vi "AutoHelper_Sequence.vi"(4 "Next Step":bool, 6 "Pass_Through_Time":dbl=-1.0 format="%33.4f", 7 "External Ready":bool=TRUE, 8 "Cancel Time Sec":dbl, 9 "Step Times Sec":dbl[](array[numeric]), 10 "Cancel":bool, 11 "Initiate":bool) -> (0 "Error":bool, 1 "Ready":bool, 2 "Seq  Active":bool, 3 "Step Number":T1=enum."Initialize", 5 "New Step":bool)   [LabVIEW 2019, in "Trajectory_Library.lvlib"]
doc: "Implements a simplified state machine similar to a mechanical / electrical drum sequencer. When the Drum Sequencer is \"Ready\" and the \"Initiate\" input becomes TRUE,, the drum sequences through its set of steps from 1 to N. After each Step is executed it is followed by a wait. During the wait the Step output indicates \"Do Nothing\". The number of Steps is determined by the number of elements in the \"Step Times\" input array. Once all the steps have been executed, the Drum Sequencer cycles bac to wait for another initiate. \n\nThere is a Cancel input that interrupts the sequence, executes the Cancel Step, performs the cancel wait, and then returns to wait for an Initiate action. \n\nIf any of the Step Times, or Cancel times are negative, or there more than 32 steps, or less than 1 step an error is signaled. The drum sequencer selects the error state and stays there.\n\nInputs:\n\nOutputs:"
uses:
  Trajectory_Library.lvlib
  Enum/DrumSequence_Step_Enum.ctl
  Enum/DrumSequence_State_Enum.ctl
  Util_GetTime_U32.vi
  Util_GetTime_U64.vi
  <vilib>/Utility/semaphor.llb/Obtain Semaphore Reference.vi
  Timer_Reset.vi
panel:
  # "Time to wait\nafter executing\nstep"
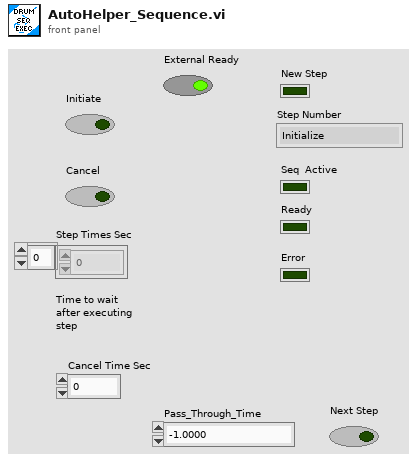
[diagram p1: front panel]
types:
  T1 = typedef "Trajectory_Library.lvlib/DrumSequence_Step_Enum.ctl" = enum16{"Do Nothing", "Step 1", "Step 2", "Step 3", "Step 4", "Step 5", "Step 6", "Step 7", "Step 8", "Step 9", "Step 10", "Step 11", "Step 12", "Step 13", "Step 14", "Step 15", "Step 16", "Step 17", "Step 18", "Step 19", "Step 20", "Step 21", "Step 22", "Step 23", "Step 24", "Step 25", "Step 26", "Step 27", "Step 28", "Step 29", "Step 30", "Step 31", "Step 32", "Cancel", "Initialize", "Error"}
  T2 = typedef "Trajectory_Library.lvlib/DrumSequence_State_Enum.ctl" = enum16{"Initialize", "Ready", "First Step", "Step Wait", "Next State", "Cancel", "Cancel Wait", "Error", "Error Loop"}
  T3 = typedef "Trajectory_Library.lvlib/TIMER.ctl" = cluster{"StartTime":dbl, "Accumulated TIme":dbl, "Running":bool, "semaphore":T4}
  T4 = typedef "Semaphore RefNum" = refnum<k1>
  T5 = typedef "DrumSequence_State_Enum.ctl" = enum16{"Initialize", "Ready", "First Step", "Step Wait", "Next State", "Cancel", "Cancel Wait", "Error", "Error Loop"}
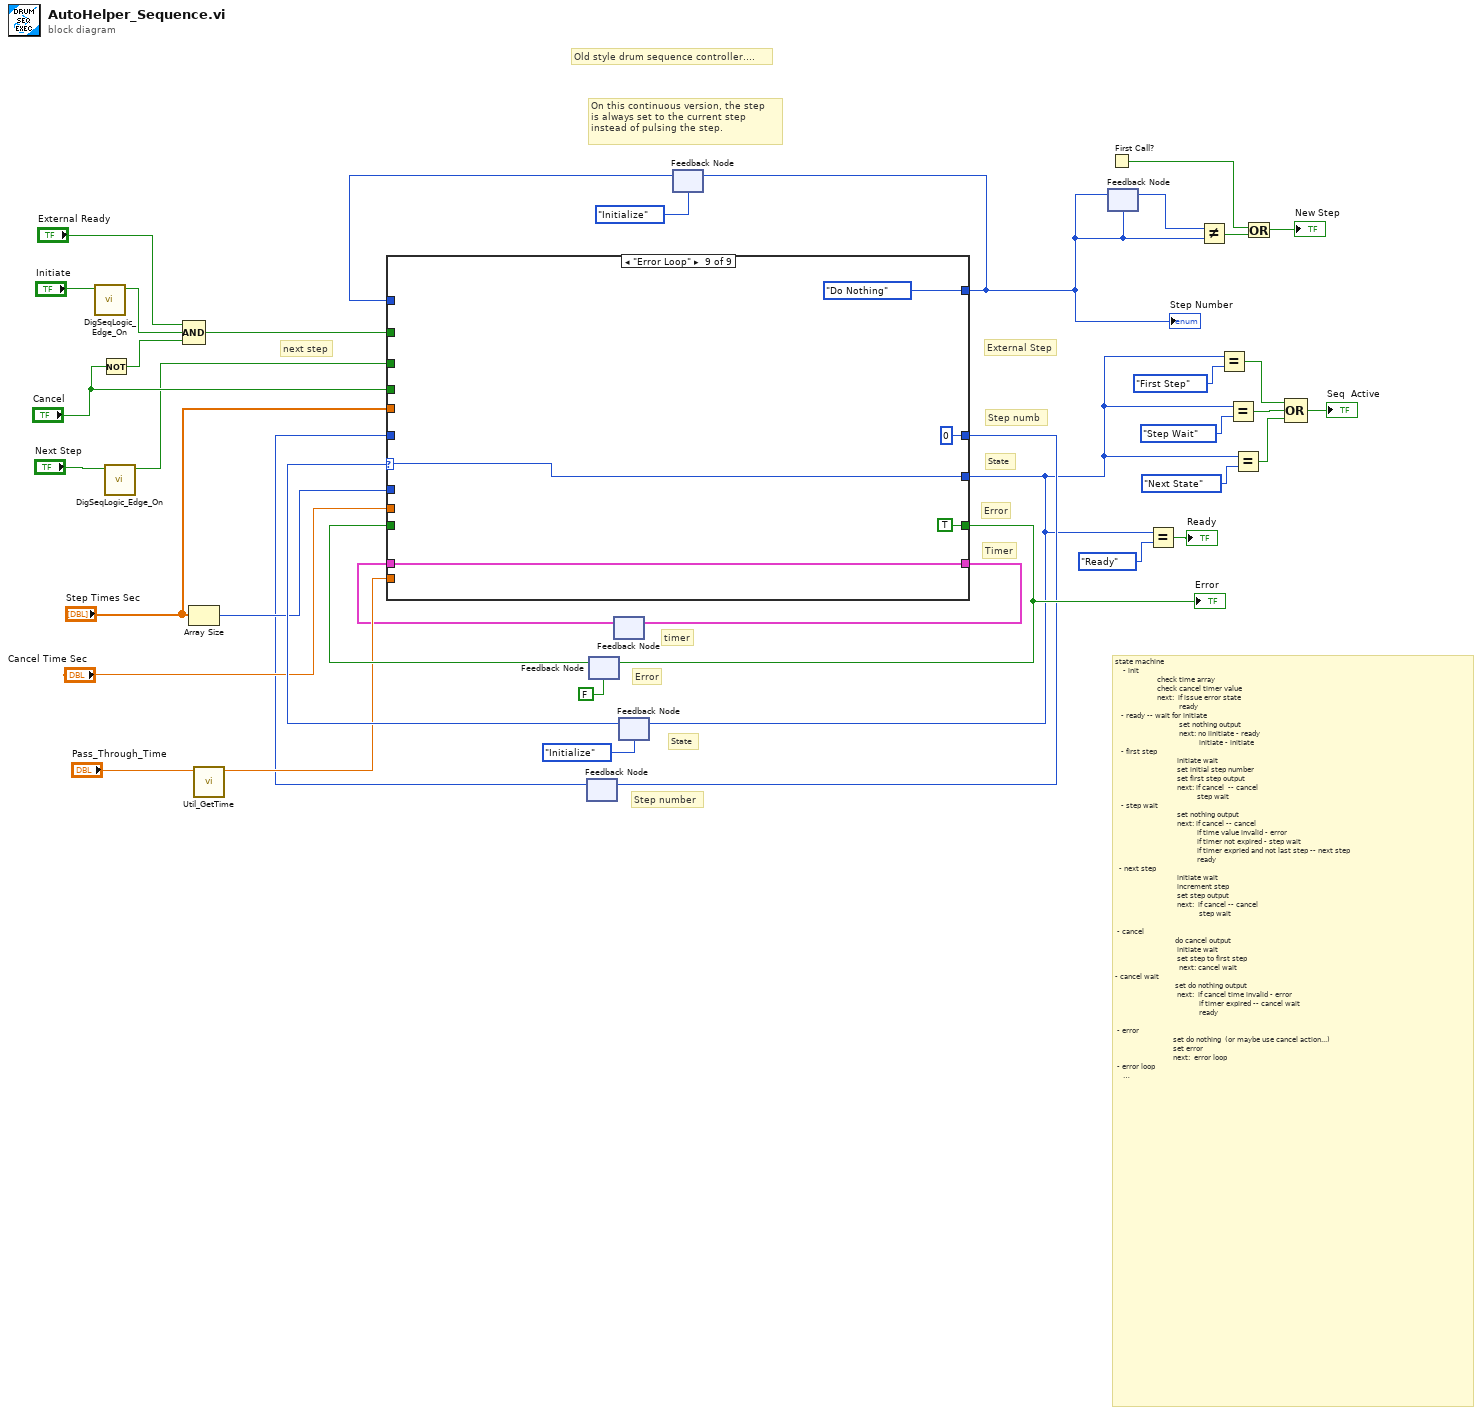
[diagram p0: block diagram]
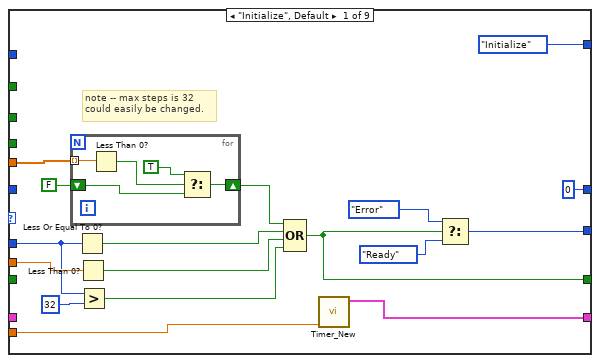
[diagram p2: hidden frame]
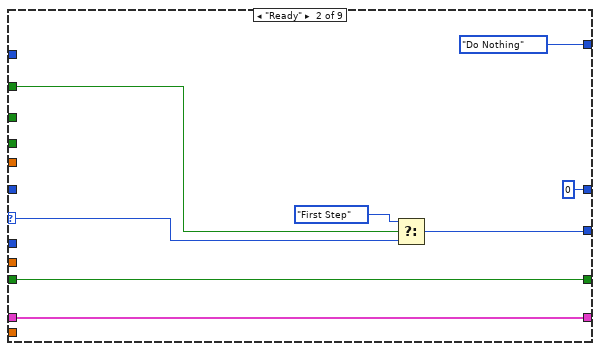
[diagram p3: hidden frame]
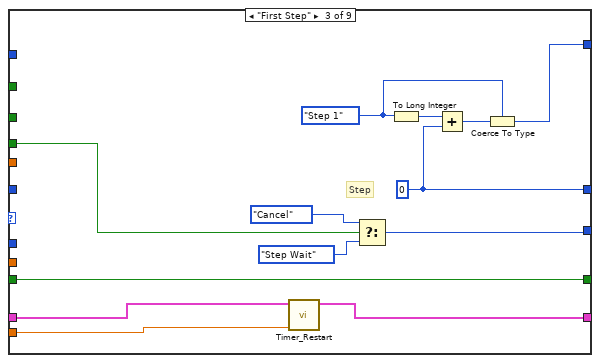
[diagram p4: hidden frame]
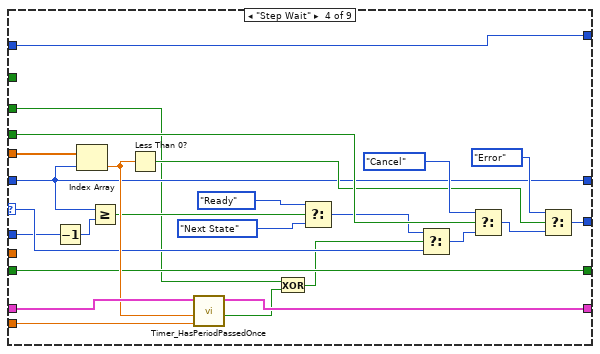
[diagram p5: hidden frame]
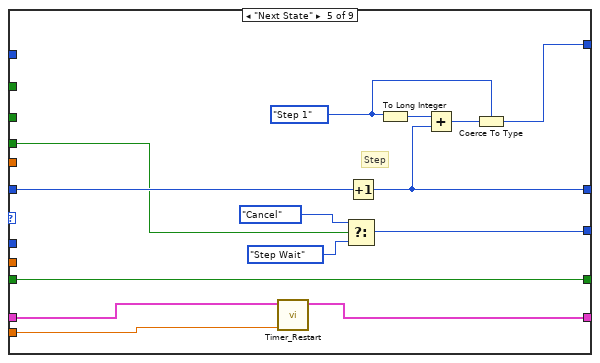
[diagram p6: hidden frame]
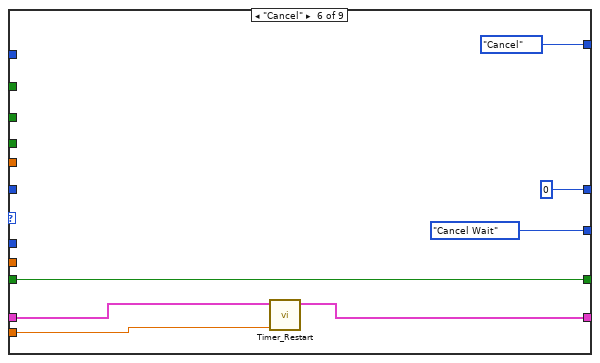
[diagram p7: hidden frame]
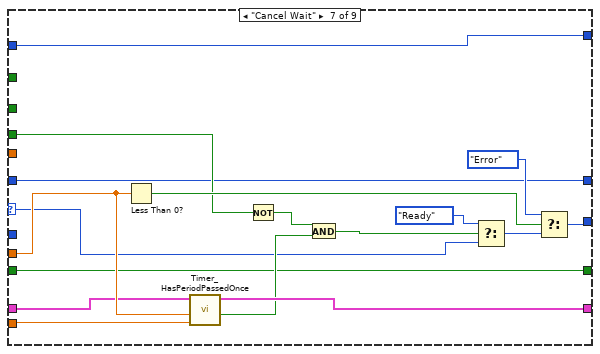
[diagram p8: hidden frame]
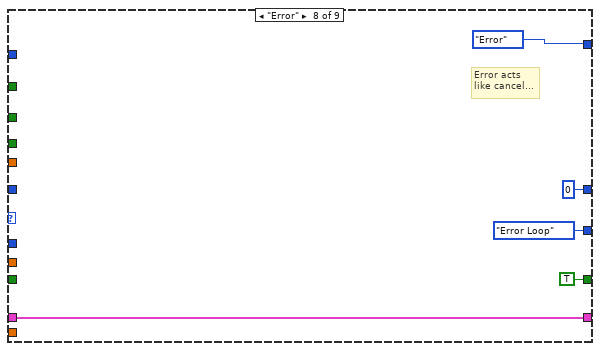
[diagram p9: hidden frame]
diagram:
  # "On this continuous version, the step\nis always set to the current step\ninstead of pulsing the step."
  # "next step"
  # "Old style drum sequence controller...."
  # "Step number"
  # "State"
  # "Step numb"
  # "timer"
  # "Timer"
  # "Error"
  # "State"
  # "External Step"
  # "Error"
  # "state machine\n    - init\n                     check time array\n                     check cancel timer value\n                     next:  if issue error state\n                                ready\n   - ready -- wait for initiate\n                                set nothing output\n                                next: no iinitiate - ready\n                                          initiate - initiate\n   - first step \n                               initiate wait\n                               set initial step number\n                               set first step output\n                               next: if cancel  -- cancel\n                                         step wait\n   - step wait \n                               set nothing output\n                               next: if cancel -- cancel\n                                         if time value invalid - error\n                                         if timer not expired - step wait\n                                         if timer expried and not last step -- next step\n                                         ready\n  - next step\n                               initiate wait\n                               increment step\n                               set step output\n                               next:  if cancel -- cancel\n                                          step wait\n\n - cancel\n                              do cancel output\n                               initiate wait\n                               set step to first step\n                                next: cancel wait\n- cancel wait\n                              set do nothing output\n                               next:  if cancel time invalid - error\n                                          if timer expired -- cancel wait\n                                          ready\n\n - error\n                             set do nothing  (or maybe use cancel action...)\n                             set error\n                             next:  error loop\n - error loop\n                             set do nothing\n                             set error\n                             next: error loop"
  n1 = call "DigSeqLogic_Edge_On.vi"("Input"="Initiate") -> ("On Edge"=w37:bool)  [unwired: 10 in]
  n2 = Not(x="Cancel") -> (.not. x?=w39:bool)
  n3 = call "DigSeqLogic_Edge_On.vi"("Input"="Next Step") -> ("On Edge"=w8:bool)  [unwired: 10 in]
  n4 = Compound Arithmetic op=AND("External Ready", w37, w39) -> (w26:bool)
  n5 = Array Size(array="Step Times Sec") -> (size(s)=w34:i32)
  n6 = call "Util_GetTime.vi"("Pass_Through_Time"="Pass_Through_Time") -> ("FPGA_Time_Seconds"=w27:dbl)  [unwired: 8 in, 2 out]
  n7 = feedback #1() -> (w20:i32)  [unwired: 1 in]
  n8 = feedback #2(FALSE) -> (w29:bool)
  n9 = feedback #3() -> (w19:T3)  [unwired: 1 in]
  n10 = feedback #4(DrumSequence_State_Enum."Initialize") -> (w35:T5)
  n11 = feedback #5(DrumSequence_Step_Enum."Initialize" ("Step Number")) -> (w1:T1)
  n12 = case shown="\"Error Loop\"" w35 {
    selector: w35 -> [_ w66 _ w90 _ _ w130 _ w154]
    tunnel: w34 -> [w44 _ _ w88 _ _ _ _ _]
    tunnel: "Step Times Sec" -> [w55 _ _ w98 _ _ _ _ _]
    tunnel: "Cancel Time Sec" -> [w54 _ _ _ _ _ w142 _ _]
    tunnel: [w50 w65 w71 w91 w112 w124 w131 TRUE TRUE] -> w30
    tunnel: w29 -> [_ w65 w71 w91 w112 w124 w131 _ _]
    tunnel: [w47 w67 w72 w95 w114 DrumSequence_State_Enum."Cancel Wait" w135 DrumSequence_State_Enum."Error Loop" w154] -> w11
    tunnel: [w46 w64 w76 w105 w109 w125 w139 w148 w152] -> w23
    tunnel: w27 -> [w45 _ w78 w106 w111 w126 w140 _ _]
    tunnel: [DrumSequence_Step_Enum."Initialize" ("Step Number") DrumSequence_Step_Enum."Do Nothing" ("Step Number") w80 w83 w115 DrumSequence_Step_Enum."Cancel" ("Step Number") w129 DrumSequence_Step_Enum."Error" ("Step Number") DrumSequence_Step_Enum."Do Nothing" ("Step Number")] -> w3
    tunnel: w26 -> [_ w69 _ _ _ _ _ _ _]
    tunnel: [0 0 w79 w92 w116 0 w133 0 0] -> w21
    tunnel: "Cancel" -> [_ _ w75 w102 w113 _ w136 _ _]
    tunnel: w20 -> [_ _ _ w92 w117 _ w133 _ _]
    tunnel: w19 -> [_ w64 w77 w107 w110 w127 w141 w148 w152]
    tunnel: w8 -> [_ _ _ w84 _ _ _ _ _]
    tunnel: w1 -> [_ _ _ w83 _ _ w129 _ _]
    frame "Initialize", Default {
      # "note -- max steps is 32\ncould easily be changed."
      n13 = for {
        shift-right: [w60] -> w53
        shift-left: FALSE -> [w59]
        tunnel: w55 -> [w61] mode=indexing
        n14 = Less Than 0?(x=w61) -> (x < 0?=w57:bool)
        n15 = Select(t=TRUE, s=w57, f=w59) -> (s? t:f=w60:bool)
      }
      n16 = Less Or Equal To 0?(x=w44) -> (x <= 0?=w52:bool)
      n17 = Less Than 0?(x=w54) -> (x < 0?=w51:bool)
      n18 = Greater?(x=w44, y=32) -> (0:w42:bool)
      n19 = Compound Arithmetic op=OR(w53, w52, w51, w42) -> (w50:bool)
      n20 = call "Timer_New.vi"("Pass_Through_Time"=w45) -> ("TIMER"=w46:T3)  [unwired: 10 in]
      n21 = Select(t=DrumSequence_State_Enum."Error", s=w50, f=DrumSequence_State_Enum."Ready") -> (s? t:f=w47:T2)
    }
    frame "Ready" {
      n22 = Select(t=DrumSequence_State_Enum."First Step", s=w69, f=w66) -> (s? t:f=w67:T5)
    }
    frame "First Step" {
      w70 = DrumSequence_Step_Enum."Step 1" ("Step Number")
      w79 = 0
      # "Step"
      n23 = call "Timer_Restart.vi"("Pass_Through_Time"=w78, "in Timer"=w77) -> ("out Timer"=w76:T3)  [unwired: 9 in]
      n24 = Select(t=DrumSequence_State_Enum."Cancel", s=w75, f=DrumSequence_State_Enum."Step Wait") -> (s? t:f=w72:T2)
      n25 = To Long Integer(number=w70) -> (32bit integer=w82:i32)
      n26 = Add(x=w82, y=w79) -> (x+y=w81:i32)
      n27 = Coerce To Type(0:w81, 1:w70) -> (2:w80:T1)
    }
    frame "Step Wait" {
      n28 = Decrement(x=w88) -> (x-1=w89:i32)
      n29 = Index Array(array=w98, index=w92) -> (element=w97:dbl)
      n30 = Greater Or Equal?(x=w92, y=w89) -> (x >= y?=w87:bool)
      n31 = Less Than 0?(x=w97) -> (x < 0?=w93:bool)
      n32 = call "Timer_HasPeriodPassedOnce.vi"("Pass_Through_Time"=w106, "Period"=w97, "in Timer"=w107) -> ("Expired"=w86:bool, "out Timer"=w105:T3)  [unwired: 6 in, 1 out]
      n33 = Exclusive Or(1:w86, 2:w84) -> (0:w85:bool)
      n34 = Select(t=DrumSequence_State_Enum."Ready", s=w87, f=DrumSequence_State_Enum."Next State") -> (s? t:f=w99:T2)
      n35 = Select(t=w99, s=w85, f=w90) -> (s? t:f=w103:T5)
      n36 = Select(t=DrumSequence_State_Enum."Cancel", s=w102, f=w103) -> (s? t:f=w94:T5)
      n37 = Select(t=DrumSequence_State_Enum."Error", s=w93, f=w94) -> (s? t:f=w95:T5)
    }
    frame "Next State" {
      w108 = DrumSequence_Step_Enum."Step 1" ("Step Number")
      # "Step"
      n38 = call "Timer_Restart.vi"("Pass_Through_Time"=w111, "in Timer"=w110) -> ("out Timer"=w109:T3)  [unwired: 9 in]
      n39 = Select(t=DrumSequence_State_Enum."Cancel", s=w113, f=DrumSequence_State_Enum."Step Wait") -> (s? t:f=w114:T2)
      n40 = Increment(x=w117) -> (x+1=w116:i32)
      n41 = To Long Integer(number=w108) -> (32bit integer=w121:i32)
      n42 = Add(x=w121, y=w116) -> (x+y=w120:i32)
      n43 = Coerce To Type(0:w120, 1:w108) -> (2:w115:T1)
    }
    frame "Cancel" {
      n44 = call "Timer_Restart.vi"("Pass_Through_Time"=w126, "in Timer"=w127) -> ("out Timer"=w125:T3)  [unwired: 9 in]
    }
    frame "Cancel Wait" {
      n45 = Less Than 0?(x=w142) -> (x < 0?=w143:bool)
      n46 = call "Timer_HasPeriodPassedOnce.vi"("Pass_Through_Time"=w140, "Period"=w142, "in Timer"=w141) -> ("Expired"=w138:bool, "out Timer"=w139:T3)  [unwired: 6 in, 1 out]
      n47 = Not(x=w136) -> (.not. x?=w137:bool)
      n48 = And(x=w137, y=w138) -> (x .and. y?=w132:bool)
      n49 = Select(t=DrumSequence_State_Enum."Ready", s=w132, f=w130) -> (s? t:f=w144:T5)
      n50 = Select(t=DrumSequence_State_Enum."Error", s=w143, f=w144) -> (s? t:f=w135:T5)
    }
    frame "Error" {
      # "Error acts\nlike cancel..."
    }
    frame "Error Loop" {
    }
  }
  "Error" <- w30
  "Step Number" <- w3
  n51 = feedback-in #1(w21) -> ()
  n52 = feedback-in #2(w30) -> ()
  n53 = feedback-in #3(w23) -> ()
  n54 = feedback-in #4(w11) -> ()
  n55 = feedback-in #5(w3) -> ()
  n56 = First Call?() -> (First Call?: T/F=w4:bool)
  n57 = feedback-in #6(w3) -> ()
  n58 = feedback #6(w3) -> (w7:T1)
  n59 = Equal?(x=w11, y=DrumSequence_State_Enum."Ready") -> (x = y?=→"Ready":bool)
  n60 = Not Equal?(x=w7, y=w3) -> (x != y?=w5:bool)
  n61 = Equal?(x=w11, y=DrumSequence_State_Enum."First Step") -> (x = y?=w15:bool)
  n62 = Equal?(x=w11, y=DrumSequence_State_Enum."Step Wait") -> (x = y?=w14:bool)
  n63 = Equal?(x=w11, y=DrumSequence_State_Enum."Next State") -> (x = y?=w13:bool)
  n64 = Or(x=w4, y=w5) -> (x .or. y?=→"New Step":bool)
  n65 = Compound Arithmetic op=OR(w15, w14, w13) -> (→"Seq  Active":bool)
